vi "Logfile.vi"(7 "Func":enum16{"写", "保存", "关闭"}(ring), 8 "error in":errorcluster caption="错误输入（无错误）", 11 "Data":string) -> (0 "error out":errorcluster caption="错误输出")   [LabVIEW 2013]
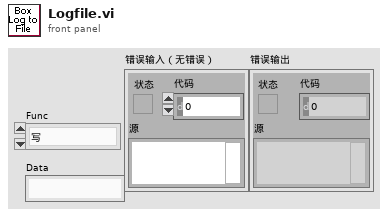
[diagram p1: front panel]
types:
  T1 = enum16{"open", "replace", "create", "open or create", "replace or create", "replace or create with confirmation"}
  T2 = typedef "LVDateTimeRec.ctl" = cluster{"秒数的小数部分":dbl, "秒":i32, "分":i32, "时":i32, "日":i32, "月":i32, "年":i32, "天数（周）":i32, "天数（年）":i32, "DST":i32}
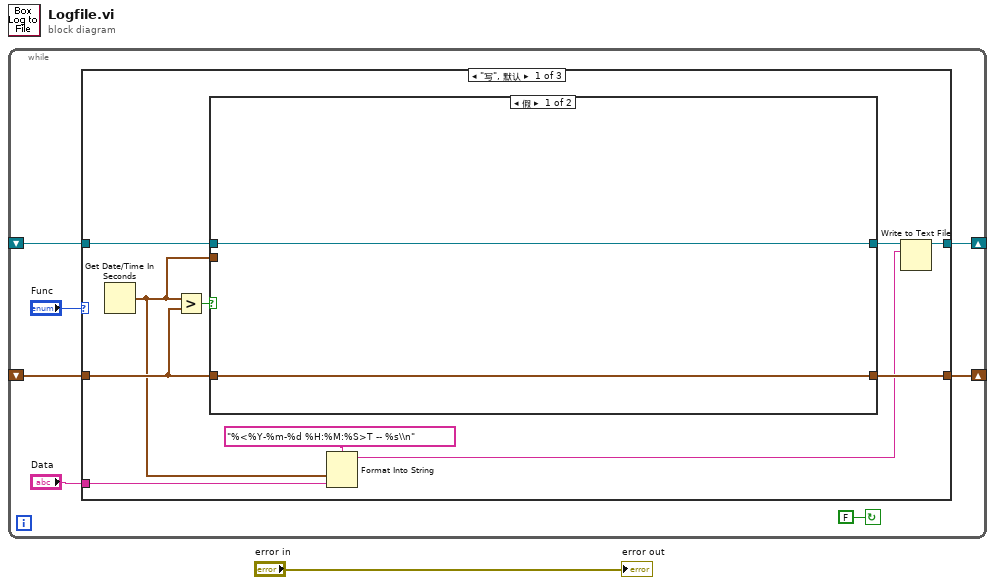
[diagram p0: block diagram]
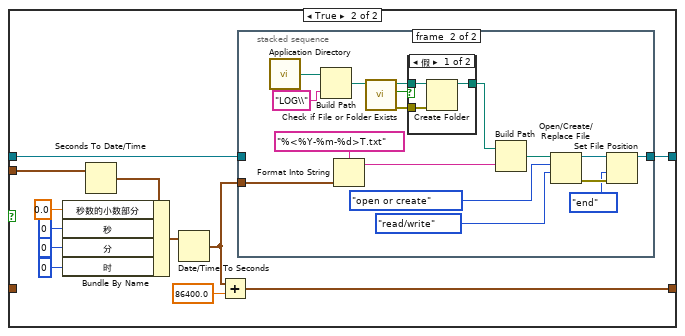
[diagram p2: hidden frame]
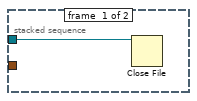
[diagram p3: hidden frame]
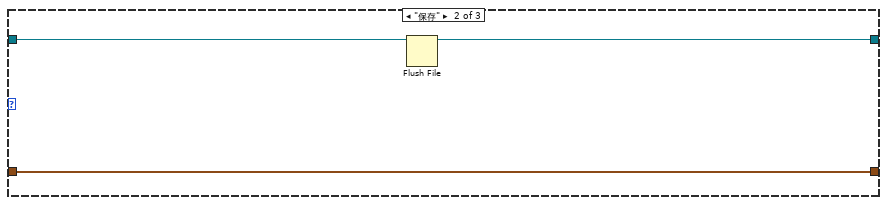
[diagram p5: hidden frame]
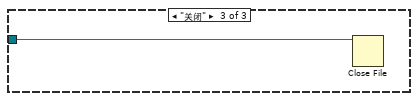
[diagram p6: hidden frame]
diagram:
  n1 = while {
    shift-right: [w8] -> _
    shift-left: _ -> [w5]
    shift-right: [w7] -> _
    shift-left: _ -> [w6]
    stop <- FALSE continue-if-true
    n2 = case shown="\"写\", 默认" "Func" {
      tunnel: [w14 w55 _] -> w8
      tunnel: [w16 w56 _] -> w7
      tunnel: w6 -> [w13 w56 _]
      tunnel: w5 -> [w17 w57 w58]
      tunnel: "Data" -> [w10 _ _]
      frame "写", Default {
        n3 = Get Date/Time In Seconds() -> (seconds since 1Jan1904=w12:timestamp)
        n4 = Greater?(x=w12, y=w13) -> (0:w18:bool)
        n5 = case shown="假" w18 {
          tunnel: [w20 w32] -> w15
          tunnel: w17 -> [w20 w31]
          tunnel: w12 -> [_ w28]
          tunnel: [w19 w30] -> w16
          tunnel: w13 -> [w19 _]
          frame False {
          }
          frame True {
            n6 = Seconds To Date/Time(time stamp (now)=w28) -> (date time rec=w27:T2)  [unwired: 1 in]
            n7 = Bundle By Name(cluster=w27, "秒数的小数部分"=0.0, "秒"=0, "分"=0, "时"=0) -> (w22:T2)
            n8 = Date/Time To Seconds(2:w22) -> (0:w21:timestamp)  [unwired: 1 in]
            n9 = Add(x=w21, y=86400.0) -> (x+y=w30:timestamp)
            n10 = stacked-sequence {
              tunnel: [_ w50] -> w32
              tunnel: w31 -> [w33 _]
              tunnel: w21 -> [_ w43]
              frame #0 {
                n11 = Close File(refnum=w33) -> ()  [unwired: 1 in, 2 out]
              }
              frame #1 {
                n12 = call <vilib>:"Application Directory.vi"() -> ("Application Directory"=w34:path)
                n13 = Build Path(base path=w34, name or relative path="LOG\\" ("初始字符串")) -> (appended path=w41:path)
                n14 = Format Into String(format string="%<%Y-%m-%d>T.txt" ("格式字符串"), w43) -> (resulting string=w35:string)  [unwired: 2 in, 1 out]
                n15 = call <vilib>:"Check if File or Folder Exists.vi"("path"=w41) -> ("error out"=w40:errorcluster, "file or folder exists?"=w38:bool, "dup path"=w39:path)  [unwired: 8 in]
                n16 = case shown="假" w38 {
                  tunnel: w40 -> [w53 _]
                  tunnel: w39 -> [w52 w54]
                  tunnel: [w51 w54] -> w36
                  frame False {
                    n17 = Create Folder(path (use dialog)=w52, error in=w53) -> (created path=w51:path)  [unwired: 1 in, 2 out]
                  }
                  frame True {
                  }
                }
                n18 = Build Path(base path=w36, name or relative path=w35) -> (appended path=w37:path)
                n19 = Open/Create/Replace File(file path (use dialog)=w37, operation (0:open)=T1."open or create" ("操作(0:open)"), access (0:read/write)=enum16{"read/write", "read-only", "write-only"}."read/write" ("权限(0:read/write)")) -> (refnum out=w47:refnum<file>, error out=w46:errorcluster)  [unwired: 3 in, 1 out]
                n20 = Set File Position(refnum=w47, from (0:start)=enum16{"start", "end", "current"}."end" ("自（0:起始）"), error in=w46) -> (refnum out=w50:refnum<file>)  [unwired: 1 in, 1 out]
              }
            }
          }
        }
        n21 = Format Into String(format string="%<%Y-%m-%d %H:%M:%S>T -- %s\\n" ("格式字符串"), w12, w10) -> (resulting string=w9:string)  [unwired: 2 in, 1 out]
        n22 = Write to Text File(file (use dialog)=w15, text=w9) -> (refnum out=w14:refnum<file>)  [unwired: 2 in, 2 out]
      }
      frame "保存" {
        n23 = Flush File(refnum=w57) -> (refnum out=w55:refnum<file>)  [unwired: 1 in, 1 out]
      }
      frame "关闭" {
        n24 = Close File(refnum=w58) -> ()  [unwired: 1 in, 2 out]
      }
    }
  }
  "error out" <- "error in"
